vi "Cosine Tapered Window.vi"   [LabVIEW 2012, in "NI_AALPro.lvlib"]
doc: "Applies a cosine tapered window to the input sequence <B>X</B>. Wire data to the <B>X</B> input to determine the polymorphic instance to use or manually select the instance."
uses:
  NI_AALPro.lvlib
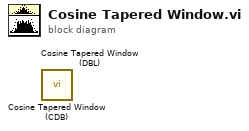
[diagram p0: block diagram]
diagram:
  n1 = call "Cosine Tapered Window (CDB).vi"() -> ()  [unwired: 10 in, 2 out]
  n2 = call "Cosine Tapered Window (DBL).vi"() -> ()  [unwired: 10 in, 2 out]
